vi "Run.vi"(8 "error in (no error)":errorcluster, 10 "Control In":T1, 11 "Assembly In":refnum<class "Assembly Run.lvclass">) -> (0 "error out":errorcluster, 2 "Control Out":T1, 3 "Assembly Out":refnum<class "Assembly Run.lvclass">)   [LabVIEW 2019, in "Assembly Run.lvclass"]
uses:
  Assembly Run.lvclass
  Controller/Controllers.ctl
  Controller/I-O/I-O.lvclass
  Controller/Dispenser/Dispenser.lvclass
  C:/Program Files (x86)/Aerotech/A3200/LabVIEW/2010/Bin/Aerotech.A3200.dll
  Program Files (x86)/Aerotech/A3200/LabVIEW/2010/Bin/Aerotech.A3200.dll
  Assembly Run.lvclass/Assembly Run.ctl
  Workspace/Fixture.lvclass
  Routine/Routine.lvclass
  Controller/Motion/A3200/A3200.lvclass
  Controller/Controller.lvclass
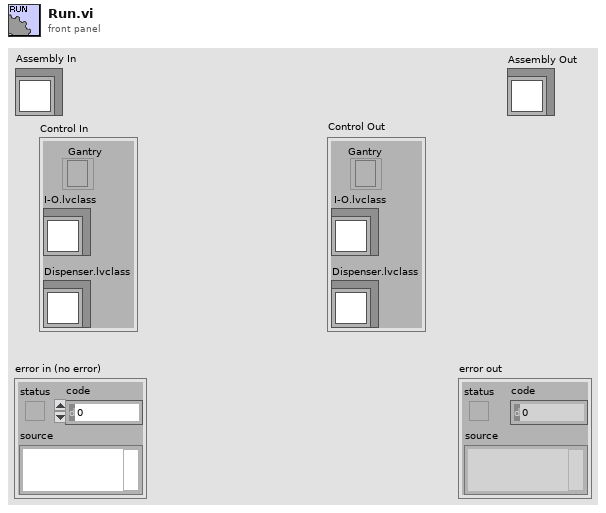
[diagram p1: front panel]
types:
  T1 = typedef "Controller.lvclass/Controllers.ctl" = cluster{"I-O.lvclass":refnum<class "I-O.lvclass">, "Dispenser.lvclass":refnum<class "Dispenser.lvclass">, "Gantry":refnum<k24>}
  T2 = typedef "Fixture.lvclass/Workspace.ctl" = cluster{"XYZTheta":dbl[], "Workspace Valve":i32, "Workspace Sensor":i32}
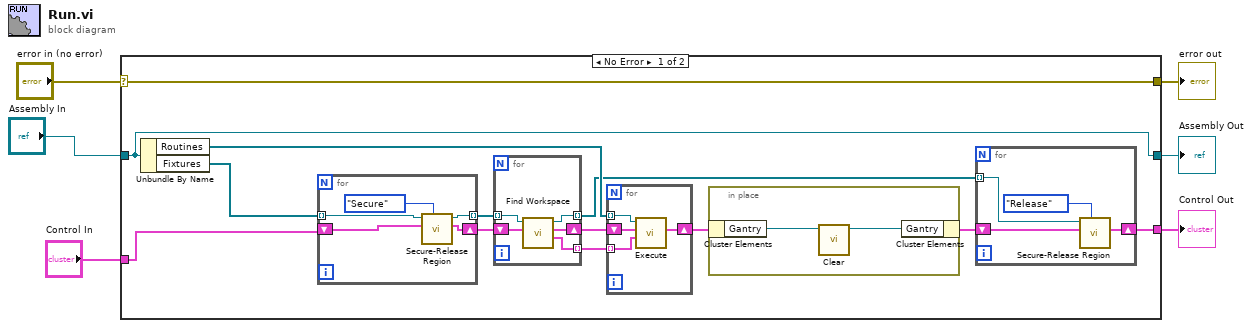
[diagram p0: block diagram]
diagram:
  n1 = case shown="No Error" "error in (no error)" {
    selector: "error in (no error)" -> [w19 w42]
    tunnel: [w19 w42] -> w5
    tunnel: "Assembly In" -> [w12 w40]
    tunnel: [w9 w41] -> w3
    tunnel: "Control In" -> [w7 w41]
    tunnel: [w12 w40] -> w1
    frame No Error {
      n2 = Unbundle By Name(w12) -> ("Routines"=w18:refnum<class "Routine.lvclass">[], "Fixtures"=w8:refnum<class "Fixture.lvclass">[])
      n3 = for {
        tunnel: [w29] -> w15 mode=indexing
        tunnel: w8 -> [w28] mode=indexing
        shift-right: [w26] -> w14
        shift-left: w7 -> [w27]
        n4 = call-dynamic "Secure-Release Region.vi"("Action"=enum16{"Secure", "Release"}."Secure", "Control In"=w27, "Fixture in"=w28) -> ("Control Out"=w26:T1, "Fixture out"=w29:refnum<class "Fixture.lvclass">)  [unwired: 6 in, 1 out]
      }
      n5 = for {
        tunnel: w15 -> [w39] mode=indexing
        tunnel: [w35] -> w17 mode=indexing
        shift-right: [w38] -> w16
        shift-left: w14 -> [w37]
        tunnel: [w36] -> w13 mode=indexing
        n6 = call-dynamic "Find Workspace.vi"("Control In"=w37, "Workspace In"=w39) -> (1:"Workspace Out"=w35:T2, "Control Out"=w38:T1, 3:"Workspace Out"=w36:refnum<class "Fixture.lvclass">)  [unwired: 6 in, 1 out]
      }
      n7 = for {
        tunnel: w18 -> [w34] mode=indexing
        tunnel: w17 -> [w33] mode=indexing
        shift-right: [w31] -> w11
        shift-left: w16 -> [w32]
        n8 = call-dynamic "Execute.vi"("Workspace"=w33, "Control In"=w32, "Routine in"=w34) -> ("Control Out"=w31:T1)  [unwired: 6 in, 2 out]
      }
      n9 = in-place {
        n10 = in-place-cluster #1(w11) -> ("Gantry"=w21:refnum<k24>)
        n11 = call "Clear.vi"("Gantry In"=w21) -> ("Gantry Out"=w20:refnum<k24>)  [unwired: 9 in, 1 out]
        n12 = in-place-cluster #1("Gantry"=w20) -> (w10:T1)
      }
      n13 = for {
        tunnel: w13 -> [w25] mode=indexing
        shift-right: [w24] -> w9
        shift-left: w10 -> [w23]
        n14 = call-dynamic "Secure-Release Region.vi"("Action"=enum16{"Secure", "Release"}."Release", "Control In"=w23, "Fixture in"=w25) -> ("Control Out"=w24:T1)  [unwired: 6 in, 2 out]
      }
    }
    frame Error {
    }
  }
  "error out" <- w5
  "Control Out" <- w3
  "Assembly Out" <- w1
